vi "ReadBase.vi"(8 "error in (no error)":errorcluster, 10 "Request Number of Message":i32, 11 "National Instruments USB-8473 Adapter Class in":refnum<class "National Instruments USB-8473 Adapter Class.lvclass">) -> (0 "error out":errorcluster, 2 "Messages":T1[](array[typedef]) {"Data" format="%02x"; "Arbitration Id" format="%03x"}, 3 "National Instruments USB-8473 Adapter Class out":refnum<class "National Instruments USB-8473 Adapter Class.lvclass">)   [LabVIEW 2011, in "National Instruments USB-8473 Adapter Class.lvclass"]
uses:
  National Instruments USB-8473 Adapter Class.lvclass
  MessageType.ctl
  Generic CAN Adapter/GenericCanAdapterClass.lvclass
  National Instruments USB-8473 Adapter Class.lvclass/National Instruments USB-8473 Adapter Class.ctl
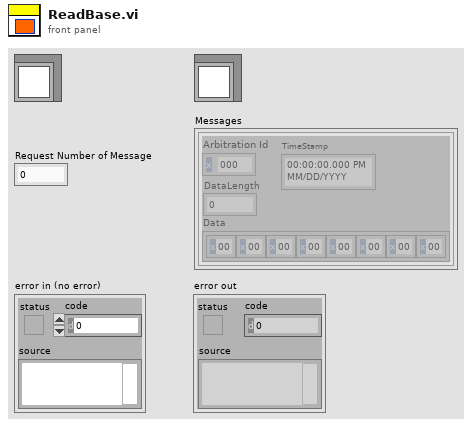
[diagram p1: front panel]
types:
  T1 = typedef "GenericCanAdapterClass.lvclass/MessageType.ctl" = cluster{"Arbitration Id":u32, "Data":u8[], "DataLength":u16, "TimeStamp":timestamp}
  T2 = typedef "xobjhandle.ctl" = u32
  T3 = typedef "CanFrameTimed.ctl" = cluster{"Timestamp":dbl, "ArbitrationId":u32, "IsRemote":u8, "DataLength":u8, "Data":u8[]}
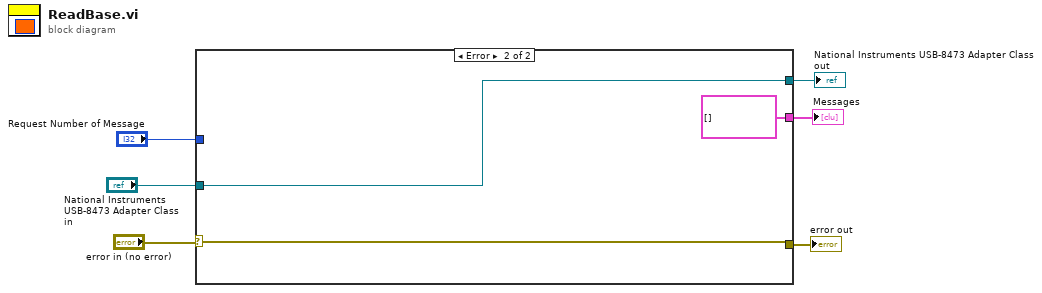
[diagram p0: block diagram]
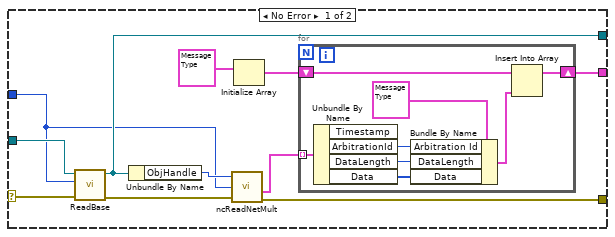
[diagram p2: hidden frame]
diagram:
  n1 = case shown="Error" "error in (no error)" {
    selector: "error in (no error)" -> [w7 w27]
    tunnel: "National Instruments USB-8473 Adapter Class in" -> [w17 w28]
    tunnel: [w15 w28] -> w5
    tunnel: "Request Number of Message" -> [w13 _]
    tunnel: [w9 T1[] []] -> w3
    tunnel: [w8 w27] -> w2
    frame No Error {
      n2 = call-parent "ReadBase.vi"("error in (no error)"=w7, "Request Number of Message"=w13, "GenericCanAdapterClass in"=w17) -> ("error out"=w16:errorcluster, "GenericCanAdapterClass out"=w15:refnum<class "National Instruments USB-8473 Adapter Class.lvclass">)  [unwired: 6 in, 1 out]
      n3 = Unbundle By Name(w15) -> ("ObjHandle"=w14:T2)
      n4 = call <vilib>:"ncReadNetMult.vi"("ObjHandle in"=w14, "Requested Number of Frames"=w13, "Error in"=w16) -> ("Data"=w10:T3[], "Error out"=w8:errorcluster)  [unwired: 2 out]
      n5 = Initialize Array(T1 {"Arbitration Id"=0, "Data"=[0, 0, 0, 0, 0, 0, 0, 0], "DataLength"=0, "TimeStamp"=timestamp(0 s since 1904-01-01)} ("MessageType")) -> (w11:T1[])  [unwired: 1 in]
      n6 = for {
        shift-right: [w24] -> w9
        shift-left: w11 -> [w25]
        tunnel: w10 -> [w18] mode=indexing
        n7 = Unbundle By Name(w18) -> ("ArbitrationId"=w22:u32, "DataLength"=w21:u8, "Data"=w20:u8[])  [unwired: 1 out]
        n8 = Bundle By Name(cluster=T1 {"Arbitration Id"=0, "Data"=[0, 0, 0, 0, 0, 0, 0, 0], "DataLength"=0, "TimeStamp"=timestamp(0 s since 1904-01-01)} ("MessageType"), "Arbitration Id"=w22, "DataLength"=w21, "Data"=w20) -> (w19:T1)
        n9 = Insert Into Array(array=w25, new element=w19) -> (w24:T1[])  [unwired: 1 in]
      }
    }
    frame Error {
    }
  }
  "error out" <- w2
  "National Instruments USB-8473 Adapter Class out" <- w5
  "Messages" <- w3
